vi "destroy.vi"(8 "error in":errorcluster, 11 "Websocket console plugin in":refnum<class "Websocket console plugin.lvclass">) -> (0 "error out":errorcluster)   [LabVIEW 2013, in "Websocket console plugin.lvclass"]
uses:
  Websocket console plugin.lvclass
  websocket user plugin.lvclass
  Websocket console plugin.lvclass/Websocket console plugin.ctl
  console UI.vi
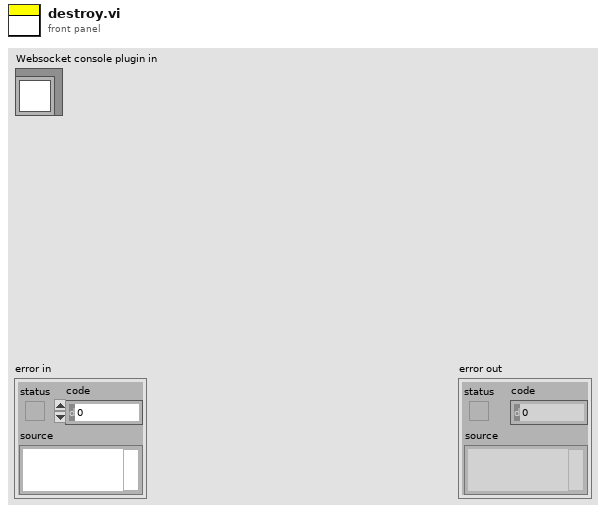
[diagram p1: front panel]
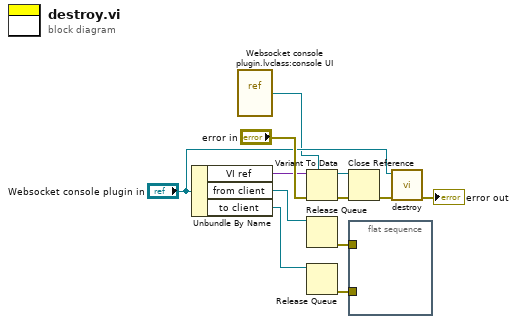
[diagram p0: block diagram]
diagram:
  n1 = Unbundle By Name("Websocket console plugin in") -> ("VI ref"=w8:variant, "from client"=w4:refnum<queue>, "to client"=w3:refnum<queue>)
  n2 = vi-ref "Websocket console plugin.lvclass:console UI.vi"() -> (w7:refnum<vi>)
  n3 = Variant To Data(error in="error in", type=w7, Variant=w8) -> (data=w5:refnum<vi>, error out=w9:errorcluster)
  n4 = Release Queue(queue=w4) -> (error out=w2:errorcluster)  [unwired: 2 in, 2 out]
  n5 = Release Queue(queue=w3) -> (error out=w1:errorcluster)  [unwired: 2 in, 2 out]
  n6 = Close Reference(reference=w5, error in (no error)=w9) -> (error out=w6:errorcluster)
  n7 = flat-sequence {
    tunnel: w2 -> [_]
    tunnel: w1 -> [_]
    frame #0 {
    }
  }
  n8 = call-parent "destroy.vi"("error in"=w6, "websocket user plugin in"="Websocket console plugin in") -> ("error out"=→"error out":errorcluster)  [unwired: 9 in]
